vi "GetNextPlayer.vi"(10 "PlayerIndex":u16) -> (2 "NewPlayerIndex":u16)   [LabVIEW 2025]
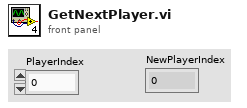
[diagram p1: front panel]
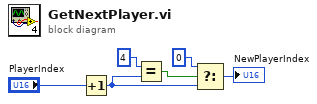
[diagram p0: block diagram]
diagram:
  n1 = Increment(x="PlayerIndex") -> (x+1=w2:u16)
  n2 = Equal?(x=4, y=w2) -> (x = y?=w3:bool)
  n3 = Select(t=0, s=w3, f=w2) -> (s? t:f=→"NewPlayerIndex":i32)
